vi "HRM-process-main.vi"(8 "error in (no error)":errorcluster, 11 "init cluster":T1) -> (0 "error out":errorcluster)   [LabVIEW 2020]
uses:
  init/HRM-init-cluster.ctl
  init/HRM-init-user_events.ctl
  init/HRM-init-start_state.ctl
  <vilib>/measure/matone.llb/Extract Single Tone Information 1 Chan.vi
  <vilib>/measure/NI_MAPro.lvlib
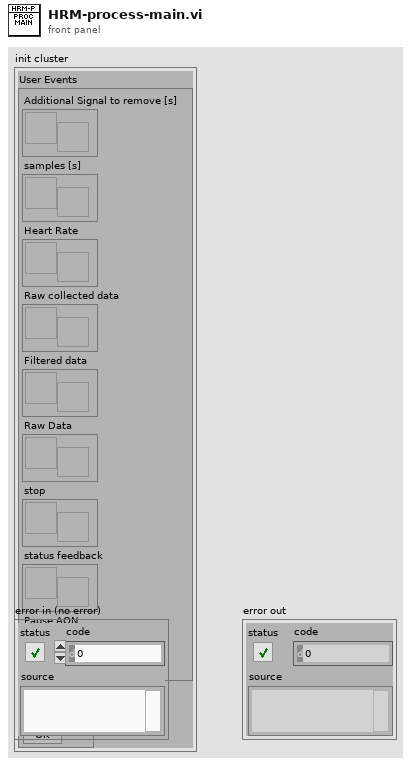
[diagram p1: front panel]
types:
  T1 = typedef "HRM-init-cluster.ctl" = cluster{"User Events":T2, "start state":T3}
  T2 = typedef "HRM-init-user_events.ctl" = cluster{"Additional Signal to remove [s]":refnum<user-event>, "samples [s]":refnum<user-event>, "Heart Rate":refnum<user-event>, "Raw collected data":refnum<user-event>, "Filtered data":refnum<user-event>, "Raw Data":refnum<user-event>, "stop":refnum<user-event>, "status feedback":refnum<user-event>, "Pause AQN":refnum<user-event>}
  T3 = typedef "HRM-init-start_state.ctl" = cluster{"Pause AQN?":bool}
  T4 = cluster{"Raw collected data":waveform(dbl), "Additional Signal to remove [s]":i32, "samples [s]":i32, "User Events":T2}
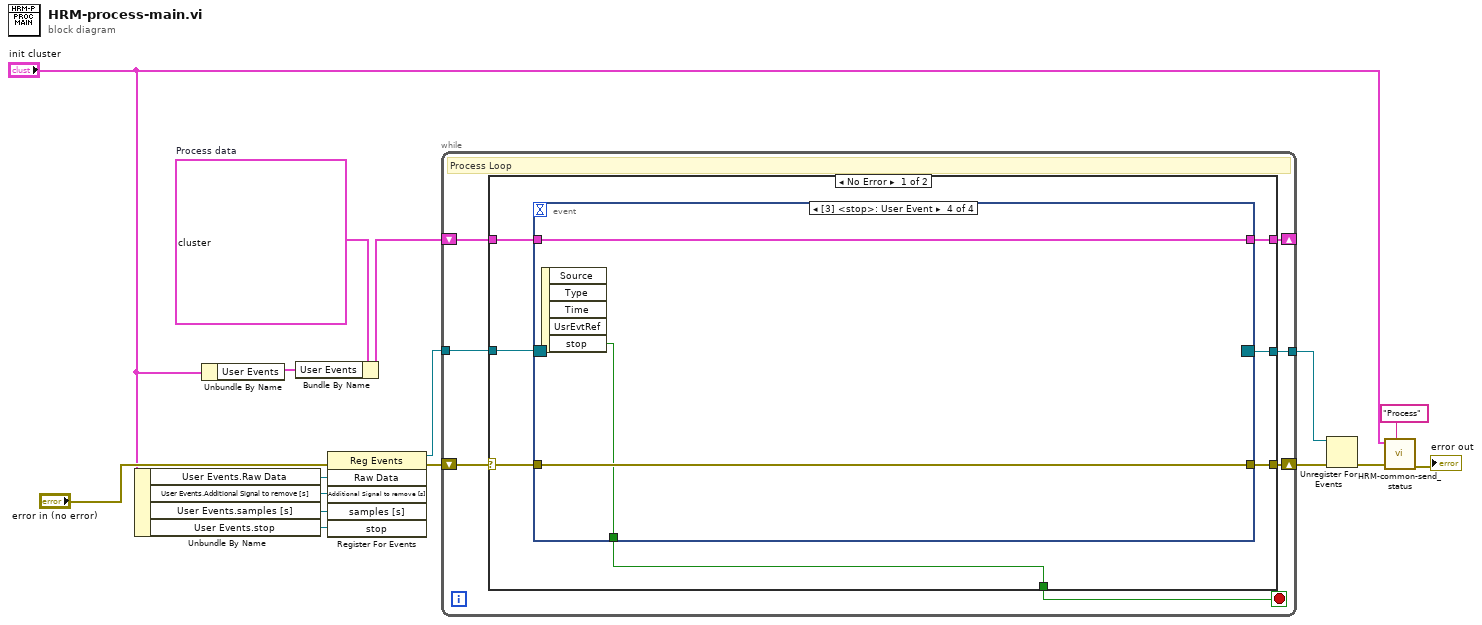
[diagram p0: block diagram]
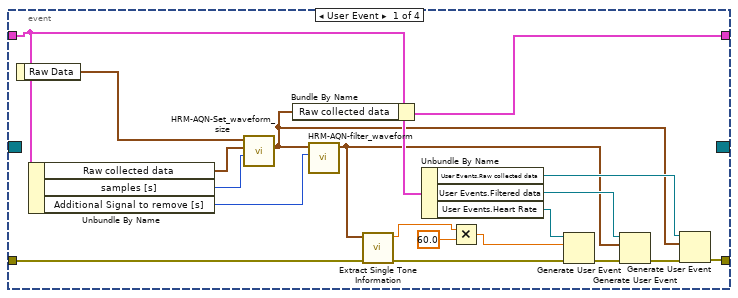
[diagram p2: hidden frame]
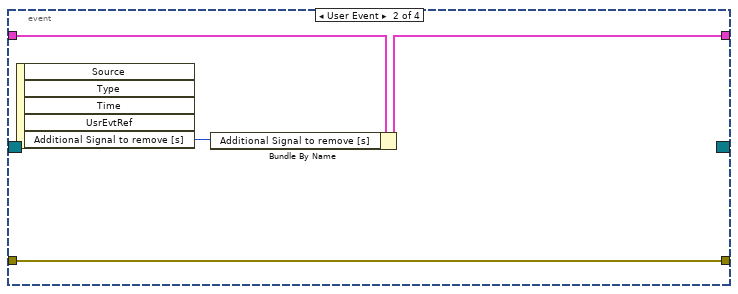
[diagram p3: hidden frame]
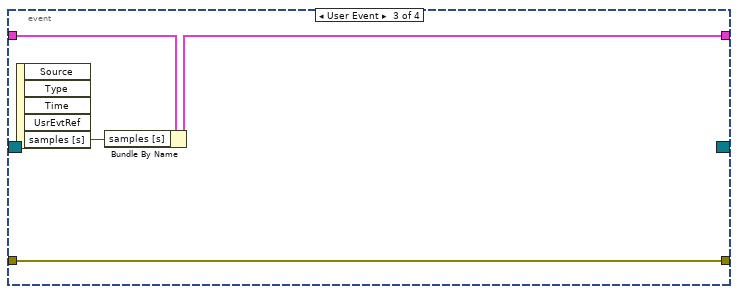
[diagram p4: hidden frame]
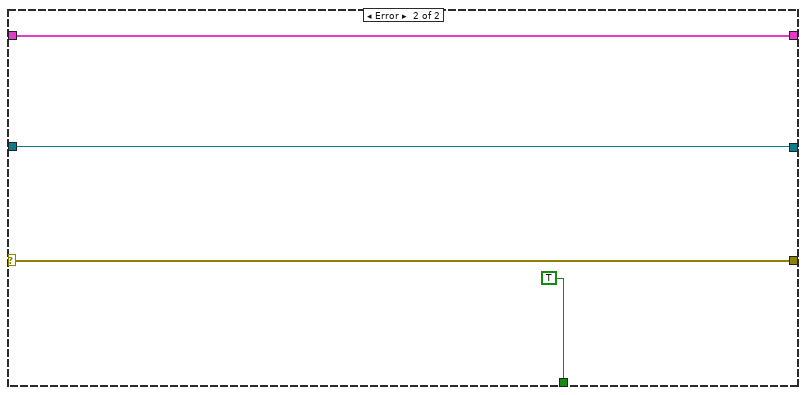
[diagram p5: hidden frame]
diagram:
  w11 = T4 {"Raw collected data"={"t0"=timestamp(0 s since 1904-01-01), "dt"=1.0, "Y"=[]}, "Additional Signal to remove [s]"=0, "samples [s]"=10, "User Events"={"Additional Signal to remove [s]"=refnum, "samples [s]"=refnum, "Heart Rate"=refnum, "Raw collected data"=refnum, "Filtered data"=refnum, "Raw Data"=refnum, "stop"=refnum, "status feedback"=refnum, "Pause AQN"=refnum}}  # Process data
  n1 = Unbundle By Name("init cluster") -> ("User Events.Raw Data"=w10:refnum<user-event>, "User Events.Additional Signal to remove [s]"=w13:refnum<user-event>, "User Events.samples [s]"=w12:refnum<user-event>, "User Events.stop"=w16:refnum<user-event>)
  n2 = Unbundle By Name("init cluster") -> ("User Events"=w15:T2)
  n3 = Bundle By Name(cluster=w11, "User Events"=w15) -> (w14:T4)
  n4 = register-events(error in="error in (no error)", w10, w13, w12, w16) -> (reference out=w5:refnum<event-registration>, error out=w7:errorcluster)  [unwired: 1 in]
  n5 = while {
    shift-right: [w22] -> w9
    shift-left: w7 -> [w23]
    shift-right: [w20] -> _
    shift-left: w14 -> [w19]
    tunnel: w5 -> [w18]
    tunnel: [w17] -> w8
    stop <- w21 stop-if-true
    # "Process Loop"
    n6 = case shown="No Error" w23 {
      selector: w23 -> [w30 w64]
      tunnel: [w29 w64] -> w22
      tunnel: [w24 TRUE] -> w21
      tunnel: [w25 w62] -> w20
      tunnel: w19 -> [w28 w62]
      tunnel: w18 -> [w27 w61]
      tunnel: [w26 w61] -> w17
      frame No Error {
        n7 = event shown="[3] <stop>: User Event" {
          selector: w27 -> [_ _ _ _]
          dyn-events: [_ _ _ _] -> w26
          timeout: _ -> [_ _ _ _]
          tunnel: w30 -> [w47 w52 w56 w60]
          tunnel: [w38 w52 w56 w60] -> w29
          tunnel: w28 -> [w45 w53 w57 w59]
          tunnel: [w37 w51 w55 w59] -> w25
          tunnel: [_ _ _ w58] -> w24
          event User Event {
            n8 = event-data() -> ("Raw Data"=w46:waveform(dbl))  [unwired: 1 in]
            n9 = Unbundle By Name(w45) -> ("Raw collected data"=w44:waveform(dbl), "samples [s]"=w43:i32, "Additional Signal to remove [s]"=w42:i32)
            n10 = call "HRM-AQN-Set_waveform_size.vi"("samples [s]"=w43, "Raw collected data"=w44, "Raw data in"=w46) -> ("Raw collected data out"=w31:waveform(dbl))  [unwired: 8 in]
            n11 = Bundle By Name(cluster=w45, "Raw collected data"=w31) -> (w37:T4)
            n12 = call "HRM-AQN-filter_waveform.vi"("Additional Signal to remove [s]"=w42, "data in"=w31) -> ("data out"=w32:waveform(dbl))  [unwired: 9 in]
            n13 = call-poly <vilib>:"Extract Single Tone Information.vi"("error in (no error)"=w47, "time signal in"=w32) -> ("error out"=w41:errorcluster, "detected frequency"=w49:dbl)  [unwired: 4 in, 4 out]
            n14 = Unbundle By Name(w37) -> ("User Events.Raw collected data"=w34:refnum<user-event>, "User Events.Filtered data"=w35:refnum<user-event>, "User Events.Heart Rate"=w36:refnum<user-event>)
            n15 = Multiply(x=w49, y=60.0) -> (x*y=w33:dbl)
            n16 = Generate User Event(user event=w36, event data cluster=w33, error in=w41) -> (error out=w40:errorcluster)  [unwired: 1 in, 1 out]
            n17 = Generate User Event(user event=w35, event data cluster=w32, error in=w40) -> (error out=w39:errorcluster)  [unwired: 1 in, 1 out]
            n18 = Generate User Event(user event=w34, event data cluster=w31, error in=w39) -> (error out=w38:errorcluster)  [unwired: 1 in, 1 out]
          }
          event User Event {
            n19 = event-data() -> ("Additional Signal to remove [s]"=w50:i32)  [unwired: 1 in, 4 out]
            n20 = Bundle By Name(cluster=w53, "Additional Signal to remove [s]"=w50) -> (w51:T4)
          }
          event User Event {
            n21 = event-data() -> ("samples [s]"=w54:i32)  [unwired: 1 in, 4 out]
            n22 = Bundle By Name(cluster=w57, "samples [s]"=w54) -> (w55:T4)
          }
          event User Event {
            n23 = event-data() -> ("stop"=w58:bool)  [unwired: 1 in, 4 out]
          }
        }
      }
      frame Error {
      }
    }
  }
  n24 = Unregister For Events(event registration refnum=w8, error in=w9) -> (error out=w4:errorcluster)
  n25 = call "HRM-common-send_status.vi"("Module name"="Process", "error in (no error)"=w4, "init cluster"="init cluster") -> ("error out"=→"error out":errorcluster)  [unwired: 8 in]
